vi "DI test MAX FPGA.vi"() -> ()   [LabVIEW 2014]
uses:
  <vilib>/rvi/Emulation/niFpgaGetClockAttributes.vi
  <vilib>/rvi/Emulation/niFpgaSctlEmulationGetInTimedLoop.vi
  <vilib>/rvi/Emulation/niFpgaEmulationReportErrorSimple.vi
  <vilib>/rvi/eio/common/nirviEmuTemplateMethod_errors.vi
  <vilib>/rvi/Emulation/niFpgaCriticalErrorInLSC.vi
  <vilib>/eio/EIONode/EIONode.xnode
panel:
  out "Mod1_31":bool
  out "Mod1_30":bool
  out "Mod1_29":bool
  out "Mod1_28":bool
  out "Mod1_22":bool
  out "Temp_SW2":bool
  out "Mod1_19":bool
  out "Mod1_18":bool
  out "H2O_PS":bool
  out "SO2_PS":bool
  out "Mod1 08":bool
  out "Mod1 07":bool
  out "SO2_GLD":bool
  out "Mod1_02":bool
  out "Mod1_01":bool
  out "Ext gas meas U":bool
  in  "stop":bool
  out "Extractor Fan":bool
  out "Door2 open":bool
  out "Door1 open":bool
  out "Temp_SW1":bool
  out "Ext gas meas D":bool
  out "CO2_PS":bool
  out "N_PS":bool
  out "CO_PS":bool
  out "HC_PS":bool
  out "AirBal_PS":bool
  out "NO_PS":bool
  out "Air_PS":bool
  out "NO_GLD":bool
  out "HC_GLD":bool
  out "CO_GLD":bool
  out "eSTOP":bool
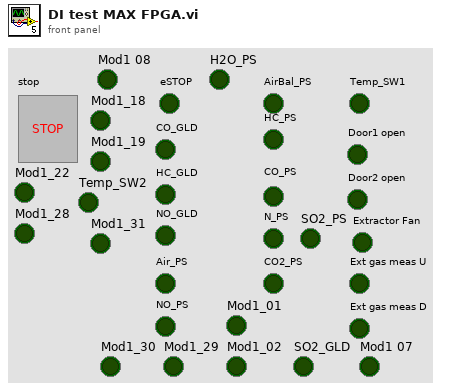
[diagram p1: front panel]
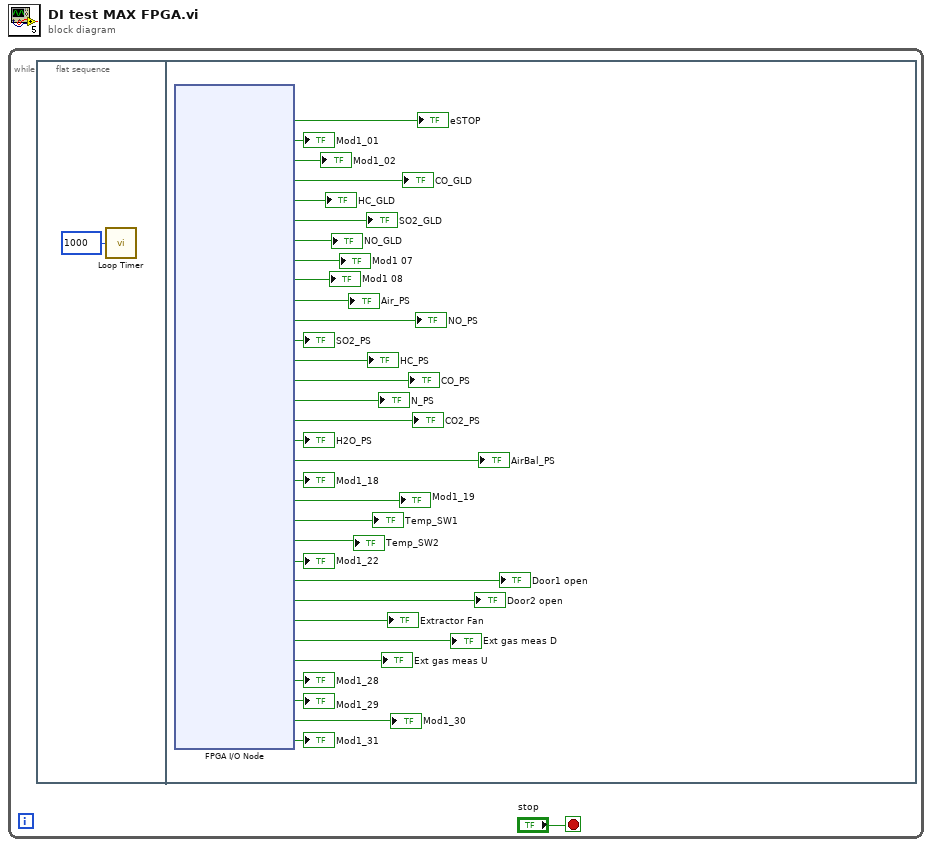
[diagram p0: block diagram]
diagram:
  n1 = while {
    stop <- "stop" stop-if-true
    n2 = flat-sequence {
      frame #0 {
        n3 = call "Loop Timer"("Count(mSec)"=u32 1000) -> ()  [unwired: 1 out]
      }
      frame #1 {
        n4 = xnode "FPGA I/O Node"() -> ("eStop"=→"eSTOP":bool, "Mod1_01"=→"Mod1_01":bool, "Mod1_02"=→"Mod1_02":bool, "CO_GLD"=→"CO_GLD":bool, "HC_GLD"=→"HC_GLD":bool, "SO2_GLD"=→"SO2_GLD":bool, "NO_GLD"=→"NO_GLD":bool, "Mod1 07"=→"Mod1 07":bool, "Mod1 08"=→"Mod1 08":bool, "Air_PS"=→"Air_PS":bool, "NO_PS"=→"NO_PS":bool, "SO2_PS"=→"SO2_PS":bool, "HC_PS"=→"HC_PS":bool, "CO_PS"=→"CO_PS":bool, "N_PS"=→"N_PS":bool, "CO2_PS"=→"CO2_PS":bool, "H2O_PS"=→"H2O_PS":bool, "AirBal_PS"=→"AirBal_PS":bool, "Mod1_18"=→"Mod1_18":bool, "Mod1_19"=→"Mod1_19":bool, "Temp_SW1"=→"Temp_SW1":bool, "Temp_SW2"=→"Temp_SW2":bool, "Mod1_22"=→"Mod1_22":bool, "DR-1_Open"=→"Door1 open":bool, "DR-2_Open"=→"Door2 open":bool, "Fan_on"=→"Extractor Fan":bool, "EGMD"=→"Ext gas meas D":bool, "EGMU"=→"Ext gas meas U":bool, "Mod1_28"=→"Mod1_28":bool, "Mod1_29"=→"Mod1_29":bool, "Mod1_30"=→"Mod1_30":bool, "Mod1_31"=→"Mod1_31":bool)  [unwired: 32 in, 32 out]
      }
    }
  }
